vi "PowerCompression.vi"() -> ()   [LabVIEW 2009]
uses:
  <vilib>/Analysis/4window.llb/windowTd.ctl
  <vilib>/measure/maspectr.llb/FFT Power Spectrum for 1 Chan.vi
  <vilib>/measure/matone.llb/Extract Single Tone Information 1 Chan.vi
  <vilib>/measure/NI_MAPro.lvlib
  <vilib>/Analysis/NI_AALPro.lvlib
panel:
  in  "Tab Control":enum32{"Configuration", "Analysis"}(tab)
  in  "Input Tone End Power (dBm)":dbl[](array[numeric])=[0.0, 0.0] format="%.2p"
  in  "Power Increment (dBm)":dbl=0.5 min=0.001
  out "Rail Voltage (+/-) in mV":dbl=10.0 format="%#_6f"
  in  "Maximum Amplifier Output Power (dBm)":dbl=-10.0
  in  "Duration (seconds)":dbl=5e-06 min=0.0
  in  "Tone Frequencies":dbl[](array[numeric])=[500000000.0, 510000000.0] format="%.2p"
  in  "Integer Degree of Nonlinearity (N) ( y(t) = x^1(t) + ...  + x^N(t) )":i32=3
  in  "Input tone Start Power (dBm)":dbl[](array[numeric])=[-40.0, -40.0] format="%.2p"
  in  "Amplifier Gain Terms (first gain term applied to linear part)":dbl[](array[numeric])=[1.0, 0.5, 0.5, 0.008, 0.016] format="%.2p"
  out "IP3 (dBm)":dbl=4.262618480732307
  out "IP2 (dBm)":dbl=6.024508123959791
  out "Total Output Power (dBm)":dbl=-10.69457410615843
  out "df (Hz)":dbl=200000.00000000003 format="%#_6p"
  out "Percent":dbl format="%#3_6f"
  out "Percent Simulation completed:":ext(slide) scale=0.0..1.0
  out "Pin vs Pout":cluster{dbl[], dbl[]}[](graph)
  out "Amplifier Output Spectrum (Frequency Domain - Magnitude)":cluster{"f0":dbl, "df":dbl, dbl[]}(graph)={"f0"=0.0, "df"=200000.00000000003, []}
  out "Amplifier Input Spectrum (Frequency Domain - Magnitude)":cluster{"f0":dbl, "df":dbl, dbl[]}(graph)={"f0"=0.0, "df"=200000.00000000003, []}
  in  "Fundamental / IMD 3":bool
  # "%"
  # "*For more information on each a control, please see the description for that control"
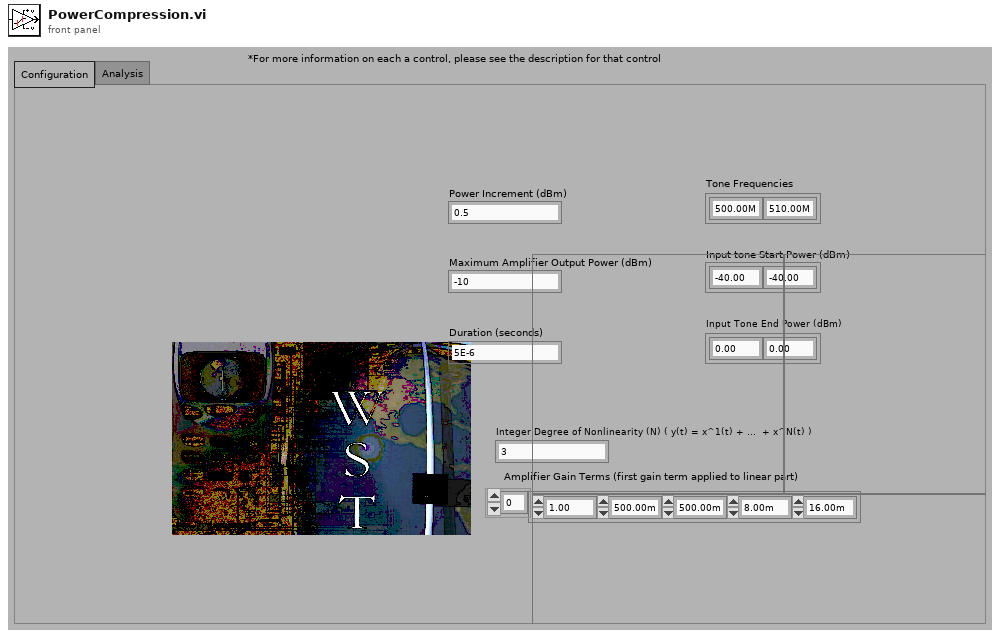
[diagram p1: front panel]
types:
  T1 = typedef "NI_AALPro.lvlib/windowTd.ctl" = u32
  T2 = cluster{"Numeric":dbl, "search (+/- % of Fsampl.)":dbl}
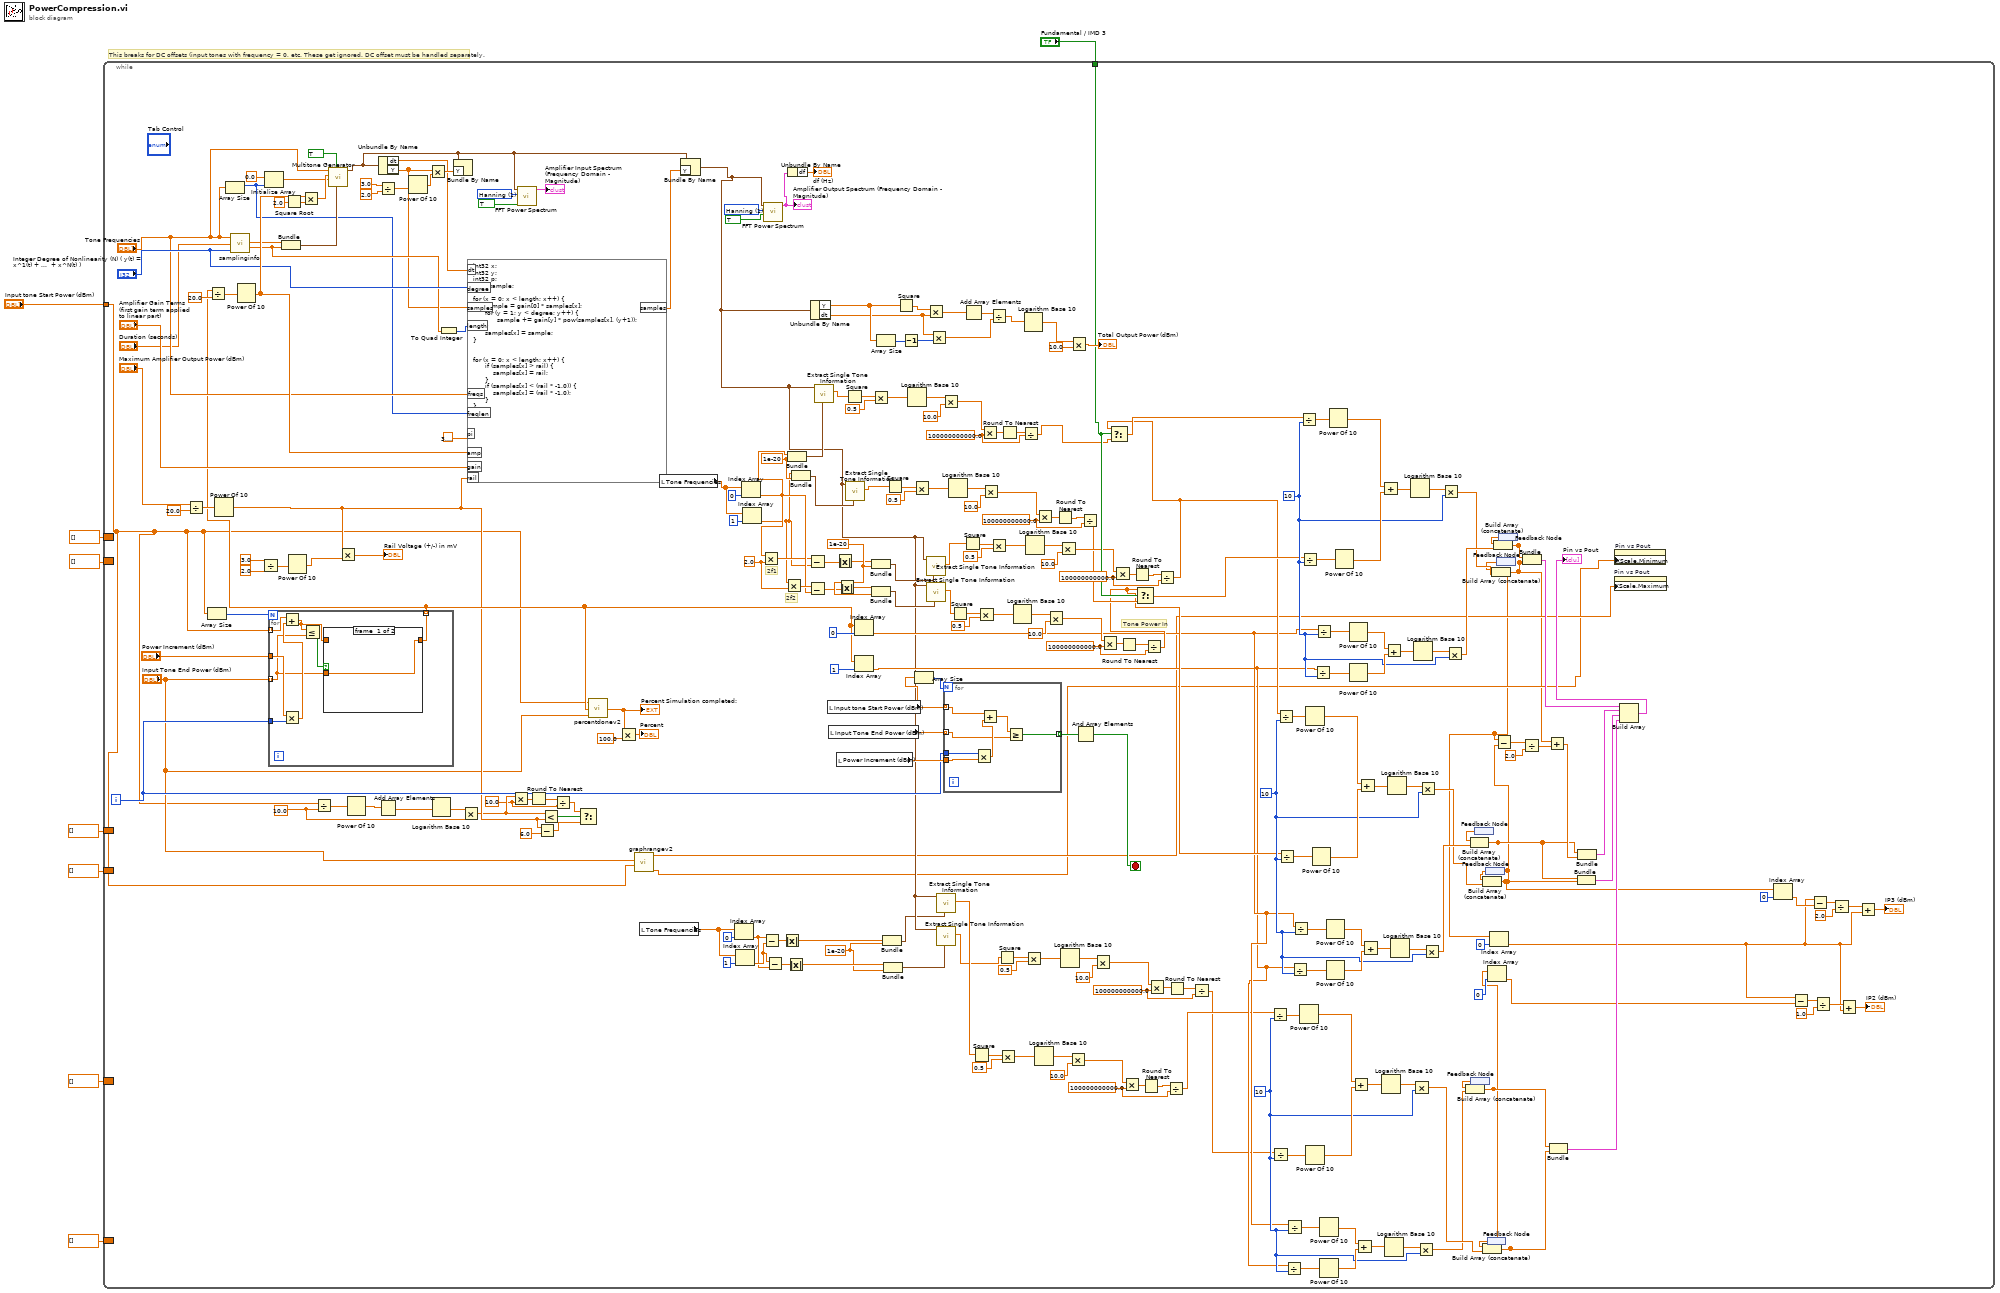
[diagram p0: block diagram]
diagram:
  # "This breaks for DC offsets (input tones with frequency = 0, etc. These get ignored. DC offset must be handled separately."
  n1 = while {
    tunnel: "Input tone Start Power (dBm)" -> [w71]
    tunnel: "Fundamental / IMD 3" -> [w142]
    border: dbl[] [] -> [_]
    border: dbl[] [] -> [_]
    border: dbl[] [] -> [_]
    border: dbl[] [] -> [_]
    border: dbl[] [] -> [_]
    border: dbl[] [] -> [_]
    i -> [w206]
    stop <- w204 stop-if-true
    w30 = 100000000000.0 ("y")
    w39 = 100000000000.0 ("y")
    w56 = 1e-20 ("search (+/- % of Fsampl.)")
    w77 = 10
    w107 = 10
    w121 = 100000000000.0 ("y")
    w131 = 100000000000.0 ("y")
    w145 = 1e-20 ("search (+/- % of Fsampl.)")
    w150 = 2.0 ("y")
    w152 = 10.0 ("y")
    w161 = 10.0 ("y")
    w172 = 10
    w212 = 100000000000.0 ("y")
    w214 = 100000000000.0 ("y")
    w233 = 1e-20 ("search (+/- % of Fsampl.)")
    w245 = T1 1 items=["Rectangle"=0, "Hanning"=1, "Hamming"=2, "Blackman-Harris"=3, "Exact Blackman"=4, "Blackman"=5, "Flat Top"=6, "4 Term B-Harris "=7, "7 Term B-Harris"=8, "Low Sidelobe"=9, "Blackman Nuttall"=11, "Triangle"=30, "Kaiser"=60, "Dolph-Chebyshev"=61, "Gaussian"=62] ("window")
    w248 = T1 1 items=["Rectangle"=0, "Hanning"=1, "Hamming"=2, "Blackman-Harris"=3, "Exact Blackman"=4, "Blackman"=5, "Flat Top"=6, "4 Term B-Harris "=7, "7 Term B-Harris"=8, "Low Sidelobe"=9, "Blackman Nuttall"=11, "Triangle"=30, "Kaiser"=60, "Dolph-Chebyshev"=61, "Gaussian"=62] ("window")
    # "2f1"
    # "2f2"
    # "Tone Power In"
    n2 = Divide(x="Maximum Amplifier Output Power (dBm)", y=20.0) -> (x/y=w255:dbl)
    n3 = Array Size(array=w71) -> (size(s)=w166:i32)
    n4 = Power Of 10(x=w255) -> (10^x=w158:dbl)
    n5 = Array Size(array="Tone Frequencies") -> (size(s)=w256:i32)
    n6 = call "samplinginfo.vi"("tone frequencies"="Tone Frequencies", "Duration"="Duration (seconds)", "Integer Degree of Nonlinearity"="Integer Degree of Nonlinearity (N) ( y(t) = x^1(t) + ...  + x^N(t) )") -> ("sampling rate"=w241:dbl, "# samples"=w259:dbl)  [unwired: 3 out]
    n7 = Divide(x=3.0, y=2.0) -> (x/y=w253:dbl)
    n8 = Initialize Array(0.0 ("element"), w256) -> (w268:dbl[])
    n9 = for {
      N: w166 -> [_]
      tunnel: w71 -> [w292] mode=indexing
      tunnel: "Input Tone End Power (dBm)" -> [w287] mode=indexing
      tunnel: "Power Increment (dBm)" -> [w291]
      tunnel: w206 -> [w290]
      tunnel: [w286] -> w188 mode=indexing
      n10 = Multiply(x=w291, y=w290) -> (x*y=w289:dbl)
      n11 = Add(x=w292, y=w289) -> (x+y=w288:dbl)
      n12 = Less Or Equal?(x=w288, y=w287) -> (x <= y?=w293:bool)
      n13 = case shown="False" w293 {
        tunnel: w288 -> [_ w295]
        tunnel: [w294 w295] -> w286
        tunnel: w287 -> [w294 _]
        frame #0 {
        }
        frame #1 {
        }
      }
    }
    n14 = Divide(x=w188, y=20.0) -> (x/y=w270:dbl[])
    n15 = Power Of 10(x=w270) -> (10^x=w271:dbl[])
    n16 = Bundle("sampling rate"=w241, "# samples"=w259) -> (w275:cluster{"sampling rate":dbl, "# samples":dbl})  [unwired: 1 in]
    n17 = Square Root(x=2.0) -> (sqrt(x)=w274:dbl)
    n18 = Power Of 10(x=w253) -> (10^x=w250:dbl)
    n19 = Multiply(x=w271, y=w274) -> (x*y=w272:dbl[])
    n20 = Divide(x=w71, y=w161) -> (x/y=w164:dbl[])
    n21 = call <vilib>:"Multitone Generator.vi"("sampling info"=w275, "reset signal"=TRUE, "tone phases"=w268, "tone amplitudes"=w272, "tone frequencies"="Tone Frequencies") -> ("signal out"=w249:waveform(dbl))  [unwired: 3 in, 3 out]
    n22 = Multiply(x=w158, y=w250) -> (x*y=→"Rail Voltage (+/-) in mV":dbl)
    n23 = Power Of 10(x=w164) -> (10^x=w163:dbl[])
    n24 = Unbundle By Name(w249) -> ("dt"=w262:dbl, "Y"=w258:dbl[])
    n25 = Divide(x=3.0, y=2.0) -> (x/y=w265:dbl)
    n26 = Add Array Elements(numeric array=w163) -> (sum=w160:dbl)
    n27 = Power Of 10(x=w265) -> (10^x=w266:dbl)
    n28 = Multiply(x=w258, y=w266) -> (x*y=w267:dbl[])
    n29 = Logarithm Base 10(1:w160) -> (0:w162:dbl)
    n30 = To Quad Integer(1:w259) -> (0:w260:i64)
    n31 = Bundle By Name(cluster=w249, "Y"=w267) -> ()  [unwired: 1 out]
    n32 = Multiply(x=w162, y=w161) -> (x*y=w153:dbl)
    n33 = formula code="int32 x;\nint32 y;\nint32 p;\nfloat sample;\n\nfor (x = 0; x < length; x++) {\n      sample = gain[0] * samples[x];\n      for (y = 1; y < degree; y++) {\n            sample += gain[y] * pow(samples[x], (y+1));  \n      }\n      samples[x] = sample;\n}\n\n\nfor (x = 0; x < length; x++) {\n      if (samples[x] > rail) {\n          samples[x] = rail;\n      }\n      if (samples[x] < (rail * -1.0)) {\n          samples[x] = (rail * -1.0);\n      }\n}"("degree"="Integer Degree of Nonlinearity (N) ( y(t) = x^1(t) + ...  + x^N(t) )", "samples"=w258, "length"=w260, "dt"=w262, "freqs"="Tone Frequencies", "freqlen"=w256, "pi"=3.141592653589793, "amp"=w271, "gain"="Amplifier Gain Terms (first gain term applied to linear part)", "rail"=w158) -> ("samples"=w239:dbl[])
    n34 = Multiply(x=w153, y=w152) -> (x*y=w155:dbl)
    n35 = call-poly <vilib>:"FFT Power Spectrum.vi"("dB On (F)"=TRUE, "window"=w248, "time signal"=w249) -> ("power spectrum"=→"Amplifier Input Spectrum (Frequency Domain - Magnitude)":cluster{"f0":dbl, "df":dbl, "magnitude":dbl[]})  [unwired: 5 in, 3 out]
    n36 = Round To Nearest(number=w155) -> (nearest integer value=w154:dbl)
    n37 = Subtract(x=w158, y=6.0) -> (x-y=w156:dbl)
    n38 = Less?(x=w153, y=w158) -> (x < y?=w159:bool)
    n39 = Divide(x=w154, y=w152) -> (x/y=w151:dbl)
    n40 = Select(t=w151, s=w159, f=w156) -> ()  [unwired: 1 out]
    n41 = call "percentdonev2.vi"("input tone end power (dBm)"="Input Tone End Power (dBm)", "Array"=w188, "input tone start power (dBm)"=w71) -> ("Numeric"=w187:dbl)
    "Percent Simulation completed:" <- w187
    n42 = Multiply(x=w187, y=100.0) -> (x*y=→"Percent":dbl)
    n43 = call "graphrangev2.vi"("input tone start power (dBm)"=w71, "input tone end power (dBm)"="Input Tone End Power (dBm)") -> ("Bottom"=w70:dbl, "Top"=w72:dbl)
    n44 = local read "Tone Frequencies"() -> (w69:dbl[])
    n45 = local read "Tone Frequencies"() -> (w236:dbl[])
    n46 = Bundle By Name(cluster=w249, "Y"=w239) -> (w74:waveform(dbl))
    n47 = Index Array(array=w69, index=0) -> (element=w61:dbl)
    n48 = Index Array(array=w69, index=1) -> (element=w62:dbl)
    n49 = Index Array(array=w236, index=0) -> (element=w148:dbl)
    n50 = Index Array(array=w236, index=1) -> (element=w146:dbl)
    n51 = Multiply(x=w148, y=w150) -> (x*y=w147:dbl)
    n52 = Subtract(x=w61, y=w62) -> (x-y=w59:dbl)
    n53 = call-poly <vilib>:"FFT Power Spectrum.vi"("dB On (F)"=TRUE, "window"=w245, "time signal"=w74) -> ("power spectrum"=w243:cluster{"f0":dbl, "df":dbl, "magnitude":dbl[]})  [unwired: 5 in, 3 out]
    "Amplifier Output Spectrum (Frequency Domain - Magnitude)" <- w243
    n54 = Subtract(x=w62, y=w61) -> (x-y=w60:dbl)
    n55 = Absolute Value(x=w59) -> (abs(x)=w58:dbl)
    n56 = Multiply(x=w146, y=w150) -> (x*y=w149:dbl)
    n57 = Absolute Value(x=w60) -> (abs(x)=w57:dbl)
    n58 = Unbundle By Name(w243) -> ("df"=→"df (Hz)":dbl)
    n59 = Bundle("Numeric"=w148, "search (+/- % of Fsampl.)"=w233) -> (w234:T2)  [unwired: 1 in]
    n60 = Bundle("Numeric"=w146, "search (+/- % of Fsampl.)"=w233) -> (w226:T2)  [unwired: 1 in]
    n61 = Subtract(x=w147, y=w146) -> (x-y=w66:dbl)
    n62 = Subtract(x=w149, y=w148) -> (x-y=w64:dbl)
    n63 = Unbundle By Name(w74) -> ("Y"=w193:dbl[], "dt"=w191:dbl)
    n64 = call-poly <vilib>:"Extract Single Tone Information.vi"("advanced search"=w234, "time signal in"=w74) -> ("detected amplitude"=w231:dbl)  [unwired: 4 in, 5 out]
    n65 = local read "Input tone Start Power (dBm)"() -> (w208:dbl[])
    n66 = local read "Input Tone End Power (dBm)"() -> (w210:dbl[])
    n67 = Absolute Value(x=w66) -> (abs(x)=w65:dbl)
    n68 = local read "Power Increment (dBm)"() -> (w209:dbl)
    n69 = Absolute Value(x=w64) -> (abs(x)=w63:dbl)
    n70 = Square(x=w231) -> (x^2=w230:dbl)
    n71 = call-poly <vilib>:"Extract Single Tone Information.vi"("advanced search"=w226, "time signal in"=w74) -> ("detected amplitude"=w220:dbl)  [unwired: 4 in, 5 out]
    n72 = Index Array(array=w188, index=0) -> (element=w76:dbl)
    n73 = Index Array(array=w188, index=1) -> (element=w75:dbl)
    n74 = Bundle(w65, "search (+/- % of Fsampl.)"=w145) -> (w144:cluster{dbl, "search (+/- % of Fsampl.)":dbl})  [unwired: 1 in]
    n75 = Bundle(w63, "search (+/- % of Fsampl.)"=w145) -> (w143:cluster{dbl, "search (+/- % of Fsampl.)":dbl})  [unwired: 1 in]
    n76 = Multiply(x=w230, y=0.5) -> (x*y=w229:dbl)
    n77 = Array Size(array=w193) -> (size(s)=w192:i32)
    n78 = Bundle(w58, "search (+/- % of Fsampl.)"=w56) -> (w54:cluster{dbl, "search (+/- % of Fsampl.)":dbl})  [unwired: 1 in]
    n79 = Bundle(w57, "search (+/- % of Fsampl.)"=w56) -> (w55:cluster{dbl, "search (+/- % of Fsampl.)":dbl})  [unwired: 1 in]
    n80 = Square(x=w220) -> (x^2=w224:dbl)
    n81 = Square(x=w193) -> (x^2=w197:dbl[])
    n82 = Decrement(x=w192) -> (x-1=w190:i32)
    n83 = Logarithm Base 10(1:w229) -> (0:w228:dbl)
    n84 = Multiply(x=w224, y=0.5) -> (x*y=w223:dbl)
    n85 = Array Size(array=w208) -> (size(s)=w207:i32)
    n86 = call-poly <vilib>:"Extract Single Tone Information.vi"("advanced search"=w144, "time signal in"=w74) -> ("detected amplitude"=w120:dbl)  [unwired: 4 in, 5 out]
    n87 = Multiply(x=w197, y=w191) -> (x*y=w196:dbl[])
    n88 = call-poly <vilib>:"Extract Single Tone Information.vi"("advanced search"=w143, "time signal in"=w74) -> ("detected amplitude"=w130:dbl)  [unwired: 4 in, 5 out]
    n89 = Multiply(x=w191, y=w190) -> (x*y=w189:dbl)
    n90 = call-poly <vilib>:"Extract Single Tone Information.vi"("advanced search"=w54, "time signal in"=w74) -> ("detected amplitude"=w29:dbl)  [unwired: 4 in, 5 out]
    n91 = call-poly <vilib>:"Extract Single Tone Information.vi"("advanced search"=w55, "time signal in"=w74) -> ("detected amplitude"=w27:dbl)  [unwired: 4 in, 5 out]
    n92 = Multiply(x=w228, y=10.0) -> (x*y=w218:dbl)
    n93 = for {
      N: w207 -> [_]
      tunnel: w208 -> [w282] mode=indexing
      tunnel: w210 -> [w280] mode=indexing
      tunnel: w209 -> [w285]
      tunnel: w206 -> [w284]
      tunnel: [w279] -> w205 mode=indexing
      n94 = Multiply(x=w284, y=w285) -> (x*y=w281:dbl)
      n95 = Add(x=w282, y=w281) -> (x+y=w283:dbl)
      n96 = Greater Or Equal?(x=w283, y=w280) -> (x >= y?=w279:bool)
    }
    n97 = Logarithm Base 10(1:w223) -> (0:w222:dbl)
    n98 = Square(x=w130) -> (x^2=w138:dbl)
    n99 = Square(x=w120) -> (x^2=w128:dbl)
    n100 = Add Array Elements(numeric array=w196) -> (sum=w195:dbl)
    n101 = Square(x=w29) -> (x^2=w37:dbl)
    n102 = Multiply(x=w138, y=0.5) -> (x*y=w137:dbl)
    n103 = Multiply(x=w218, y=w212) -> (x*y=w217:dbl)
    n104 = Multiply(x=w222, y=10.0) -> (x*y=w219:dbl)
    n105 = Divide(x=w195, y=w189) -> (x/y=w194:dbl)
    n106 = Multiply(x=w128, y=0.5) -> (x*y=w127:dbl)
    n107 = Square(x=w27) -> (x^2=w46:dbl)
    n108 = Multiply(x=w37, y=0.5) -> (x*y=w36:dbl)
    n109 = Round To Nearest(number=w217) -> (nearest integer value=w213:dbl)
    n110 = Logarithm Base 10(1:w137) -> (0:w136:dbl)
    n111 = Divide(x=w213, y=w212) -> (x/y=w104:dbl)
    n112 = Logarithm Base 10(1:w194) -> (0:w200:dbl)
    n113 = Multiply(x=w46, y=0.5) -> (x*y=w45:dbl)
    n114 = Logarithm Base 10(1:w127) -> (0:w126:dbl)
    n115 = Logarithm Base 10(1:w36) -> (0:w35:dbl)
    n116 = Multiply(x=w219, y=w214) -> (x*y=w216:dbl)
    n117 = Multiply(x=w136, y=10.0) -> (x*y=w134:dbl)
    n118 = Round To Nearest(number=w216) -> (nearest integer value=w215:dbl)
    n119 = Multiply(x=w126, y=10.0) -> (x*y=w124:dbl)
    n120 = Logarithm Base 10(1:w45) -> (0:w44:dbl)
    n121 = Multiply(x=w35, y=10.0) -> (x*y=w33:dbl)
    n122 = Multiply(x=w200, y=10.0) -> (x*y=→"Total Output Power (dBm)":dbl)
    n123 = And Array Elements(Boolean array=w205) -> (logical AND=w204:bool)
    n124 = Divide(x=w215, y=w214) -> (x/y=w103:dbl)
    n125 = Multiply(x=w44, y=10.0) -> (x*y=w42:dbl)
    n126 = Multiply(x=w134, y=w131) -> (x*y=w133:dbl)
    n127 = Multiply(x=w124, y=w121) -> (x*y=w123:dbl)
    n128 = Round To Nearest(number=w133) -> (nearest integer value=w132:dbl)
    n129 = Multiply(x=w33, y=w30) -> (x*y=w32:dbl)
    n130 = Round To Nearest(number=w123) -> (nearest integer value=w122:dbl)
    n131 = Round To Nearest(number=w32) -> (nearest integer value=w31:dbl)
    n132 = Divide(x=w132, y=w131) -> (x/y=w93:dbl)
    n133 = Select(t=w93, s=w142, f=w103) -> (s? t:f=w141:dbl)
    n134 = Multiply(x=w42, y=w39) -> (x*y=w41:dbl)
    n135 = Divide(x=w122, y=w121) -> (x/y=w92:dbl)
    n136 = Select(t=w92, s=w142, f=w104) -> (s? t:f=w140:dbl)
    n137 = Divide(x=w31, y=w30) -> (x/y=w28:dbl)
    n138 = Round To Nearest(number=w41) -> (nearest integer value=w40:dbl)
    n139 = Divide(x=w40, y=w39) -> (x/y=w26:dbl)
    n140 = Divide(x=w28, y=w77) -> (x/y=w78:dbl)
    n141 = Divide(x=w26, y=w77) -> (x/y=w79:dbl)
    n142 = Divide(x=w92, y=w107) -> (x/y=w108:dbl)
    n143 = Divide(x=w93, y=w107) -> (x/y=w109:dbl)
    n144 = Divide(x=w75, y=w77) -> (x/y=w81:dbl)
    n145 = Divide(x=w76, y=w77) -> (x/y=w80:dbl)
    n146 = Divide(x=w75, y=w107) -> (x/y=w111:dbl)
    n147 = Divide(x=w76, y=w107) -> (x/y=w110:dbl)
    n148 = Divide(x=w140, y=w172) -> (x/y=w173:dbl)
    n149 = Power Of 10(x=w78) -> (10^x=w84:dbl)
    n150 = Divide(x=w141, y=w172) -> (x/y=w174:dbl)
    n151 = Power Of 10(x=w108) -> (10^x=w114:dbl)
    n152 = Power Of 10(x=w79) -> (10^x=w85:dbl)
    n153 = Power Of 10(x=w109) -> (10^x=w115:dbl)
    n154 = Divide(x=w75, y=w172) -> (x/y=w176:dbl)
    n155 = Divide(x=w76, y=w172) -> (x/y=w175:dbl)
    n156 = Power Of 10(x=w80) -> (10^x=w82:dbl)
    n157 = Power Of 10(x=w81) -> (10^x=w83:dbl)
    n158 = Power Of 10(x=w110) -> (10^x=w112:dbl)
    n159 = Power Of 10(x=w111) -> (10^x=w113:dbl)
    n160 = Power Of 10(x=w173) -> (10^x=w179:dbl)
    n161 = Power Of 10(x=w174) -> (10^x=w180:dbl)
    n162 = Power Of 10(x=w175) -> (10^x=w177:dbl)
    n163 = Power Of 10(x=w176) -> (10^x=w178:dbl)
    n164 = Add(x=w84, y=w85) -> (x+y=w86:dbl)
    n165 = Add(x=w82, y=w83) -> (x+y=w87:dbl)
    n166 = Add(x=w114, y=w115) -> (x+y=w116:dbl)
    n167 = Add(x=w112, y=w113) -> (x+y=w117:dbl)
    n168 = Add(x=w179, y=w180) -> (x+y=w181:dbl)
    n169 = Logarithm Base 10(1:w86) -> (0:w88:dbl)
    n170 = Add(x=w177, y=w178) -> (x+y=w182:dbl)
    n171 = Logarithm Base 10(1:w87) -> (0:w89:dbl)
    n172 = Logarithm Base 10(1:w116) -> (0:w118:dbl)
    n173 = Logarithm Base 10(1:w117) -> (0:w119:dbl)
    n174 = Logarithm Base 10(1:w181) -> (0:w183:dbl)
    n175 = Multiply(x=w88, y=w77) -> (x*y=w51:dbl)
    n176 = Logarithm Base 10(1:w182) -> (0:w184:dbl)
    n177 = Multiply(x=w89, y=w77) -> (x*y=w50:dbl)
    n178 = Multiply(x=w118, y=w107) -> (x*y=w105:dbl)
    n179 = Multiply(x=w119, y=w107) -> (x*y=w106:dbl)
    n180 = Multiply(x=w183, y=w172) -> (x*y=w168:dbl)
    n181 = Multiply(x=w184, y=w172) -> (x*y=w171:dbl)
    n182 = feedback #1() -> (w53:dbl[])
    n183 = Build Array (concatenate)(w53, w50) -> (w49:dbl[])
    n184 = feedback #2() -> (w94:dbl[])
    n185 = Build Array (concatenate)(w94, w106) -> (w91:dbl[])
    n186 = feedback #3() -> (w95:dbl[])
    n187 = Build Array (concatenate)(w95, w105) -> (w15:dbl[])
    n188 = feedback #4() -> (w52:dbl[])
    n189 = Build Array (concatenate)(w52, w51) -> (w19:dbl[])
    n190 = Index Array(array=w19, index=0) -> (element=w17:dbl)
    n191 = feedback #5() -> (w167:dbl[])
    n192 = Build Array (concatenate)(w167, w168) -> (w21:dbl[])
    n193 = Index Array(array=w21, index=0) -> (element=w9:dbl)
    n194 = Subtract(x=w21, y=w15) -> (x-y=w102:dbl[])
    n195 = feedback #6() -> (w170:dbl[])
    n196 = Build Array (concatenate)(w170, w171) -> (w169:dbl[])
    n197 = Bundle(w169, w21) -> (w98:cluster{dbl[], dbl[]})  [unwired: 1 in]
    n198 = Divide(x=w102, y=2.0) -> (x/y=w100:dbl[])
    n199 = Add(x=w21, y=w100) -> (x+y=w99:dbl[])
    n200 = Bundle(w49, w19) -> (w48:cluster{dbl[], dbl[]})  [unwired: 1 in]
    n201 = Bundle(w91, w15) -> (w90:cluster{dbl[], dbl[]})  [unwired: 1 in]
    n202 = Bundle(w91, w99) -> (w97:cluster{dbl[], dbl[]})  [unwired: 1 in]
    n203 = property on="Pin vs Pout" class="XYGraph (strict)"("XScale.Maximum"=w72) -> ()  [unwired: 2 in, 2 out]
    n204 = property on="Pin vs Pout" class="XYGraph (strict)"("XScale.Minimum"=w70) -> ()  [unwired: 2 in, 2 out]
    n205 = Build Array(w98, w97, w90, w48) -> (→"Pin vs Pout":cluster{dbl[], dbl[]}[])
    n206 = Index Array(array=w15, index=0) -> (element=w10:dbl)
    n207 = Subtract(x=w9, y=w17) -> (x-y=w24:dbl)
    n208 = Subtract(x=w9, y=w10) -> (x-y=w13:dbl)
    n209 = Divide(x=w24, y=1.0) -> (x/y=w23:dbl)
    n210 = Divide(x=w13, y=2.0) -> (x/y=w12:dbl)
    n211 = Add(x=w23, y=w9) -> (x+y=→"IP2 (dBm)":dbl)
    n212 = Add(x=w12, y=w9) -> (x+y=→"IP3 (dBm)":dbl)
  }
